vi "_closeLog.vi"(8 "error in (no error)":errorcluster, 11 "SkynetCompiler in":refnum<class "LVAutomationListener.lvclass">) -> (0 "error out":errorcluster, 3 "SkynetCompiler out":refnum<class "LVAutomationListener.lvclass">)   [LabVIEW 2013, in "LVAutomationListener.lvlib" / "LVAutomationListener.lvclass"]
uses:
  LVAutomationListener.lvclass
  LVAutomationListener.lvclass/LVAutomationListener.ctl
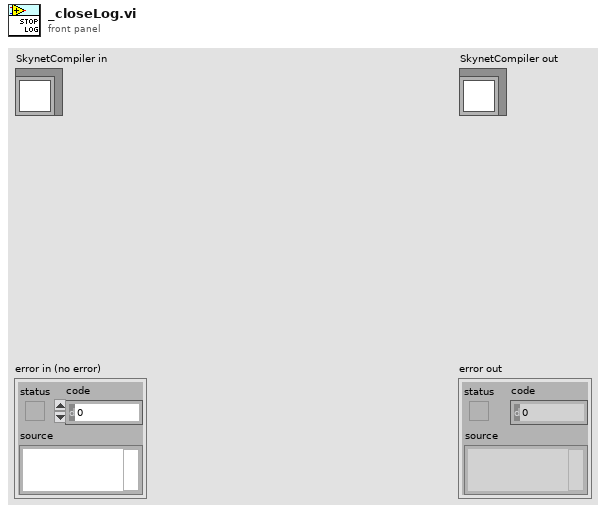
[diagram p1: front panel]
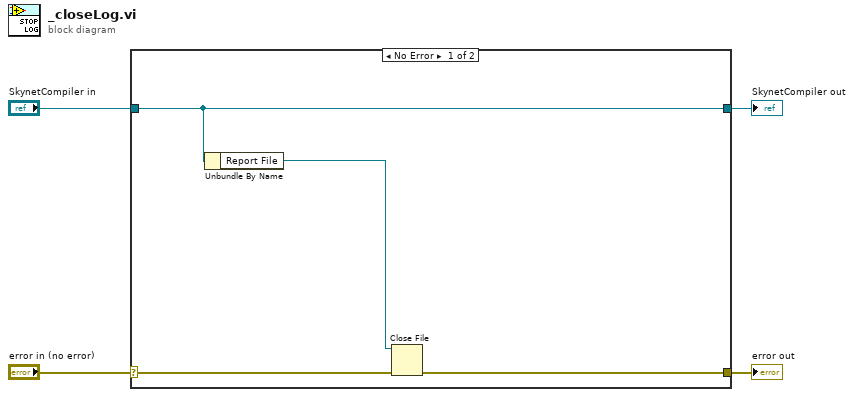
[diagram p0: block diagram]
diagram:
  n1 = case shown="No Error" "error in (no error)" {
    selector: "error in (no error)" -> [w7 w10]
    tunnel: [w5 w10] -> w3
    tunnel: [w8 w9] -> w1
    tunnel: "SkynetCompiler in" -> [w8 w9]
    frame No Error {
      n2 = Unbundle By Name(w8) -> ("Report File"=w6:refnum<file>)
      n3 = Close File(refnum=w6, error in=w7) -> (error out=w5:errorcluster)  [unwired: 1 out]
    }
    frame Error {
    }
  }
  "error out" <- w3
  "SkynetCompiler out" <- w1
